vi "Measurement Logic.vi"() -> ()   [LabVIEW 2021, in "Line Regulation_PMIC.lvlib"]
uses:
  Line Regulation_PMIC.lvlib
  Measurement Configuration.ctl
  Measurement Results.ctl
  <vilib>/Plug-In SDKs/Measurements/Measure Call Context/Measure Call Context.lvclass
  <instrlib>/niDCPower/nidcpower.llb/niDCPower Sense.ctl
  <instrlib>/niDCPower/nidcpower.llb/niDCPower Source Mode.ctl
  <instrlib>/niDCPower/nidcpower.llb/niDCPower Wait For Event - Event.ctl
  <instrlib>/niDCPower/nidcpower.llb/niDCPower Output Function.ctl
  <instrlib>/niDCPower/nidcpower.llb/niDCPower Sequence Attribute Type.ctl
  <instrlib>/niDCPower/nidcpower.llb/niDCPower Get Channel Name From String.vi
  <instrlib>/niDCPower/nidcpower.llb/niDCPower Create Advanced Sequence Step With Channels.vi
  <instrlib>/niDCPower/nidcpower.llb/niDCPower Configure Digital Edge Source Trigger With Channels.vi
  <instrlib>/niDCPower/nidcpower.llb/niDCPower Configure Digital Edge Measure Trigger With Channels.vi
panel:
  out "measure call context out":refnum<class "Measure Call Context.lvclass">
  in  "measure call context in":refnum<class "Measure Call Context.lvclass">
  out "measurement results":T1
  in  "measurement configuration":T2={"Mode of operation"=enum."Perform measurement", "DUT setup time"=1.0, "Source delay"=0.005, "Aperture time"=0.005, "Nominal output voltage"=3.3, "Source resource name"="", "Source current limit"=25.0, "Source maximum power"=300.0, "Source sweep type"="Logarithmic", "Source start voltage"=6.0, "Source stop voltage"=20.0, "Source voltage sweep points/points per decade"=4, "Load resource name"="", "Load voltage limit range"=6.0, "Load current level"=0.1}
  out "error out":errorcluster
  in  "error in":errorcluster
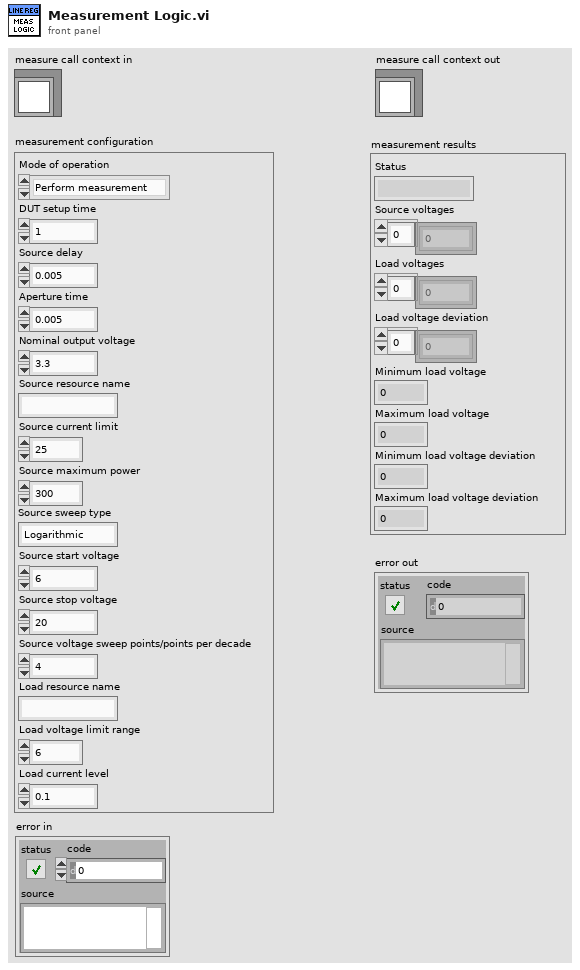
[diagram p1: front panel]
types:
  T1 = typedef "Line Regulation_PMIC.lvlib/Measurement Results.ctl" = cluster{"Status":string, "Source voltages":dbl[], "Load voltages":dbl[], "Load voltage deviation":dbl[], "Minimum load voltage":dbl, "Maximum load voltage":dbl, "Minimum load voltage deviation":dbl, "Maximum load voltage deviation":dbl}
  T2 = typedef "Line Regulation_PMIC.lvlib/Measurement Configuration.ctl" = cluster{"Mode of operation":enum32{"Power on the DUT", "Perform measurement", "Power off the DUT"}, "DUT setup time":dbl, "Source delay":dbl, "Aperture time":dbl, "Nominal output voltage":dbl, "Source resource name":string, "Source current limit":dbl, "Source maximum power":dbl, "Source sweep type":string, "Source start voltage":dbl, "Source stop voltage":dbl, "Source voltage sweep points/points per decade":i32, "Load resource name":string, "Load voltage limit range":dbl, "Load current level":dbl}
  T3 = cluster{"Voltage values":dbl[], "Source out":refnum<k15>, "Source channel name":string, "Load out":refnum<k15>, "Load channel name":string, "Source terminal name":string, "Measure terminal name":string, "Source sequence name":string, "Measurement Results":T1}
  T4 = enum32{"Power on the DUT", "Perform measurement", "Power off the DUT"}
  T5 = typedef "niDCPower Wait For Event - Event.ctl" = i32
  T6 = typedef "niDCPower Source Mode.ctl" = i32
  T7 = typedef "niDCPower Sense.ctl" = i32
  T8 = typedef "niDCPower Sequence Attribute Type.ctl" = i32
  T9 = typedef "niDCPower Output Function.ctl" = i32
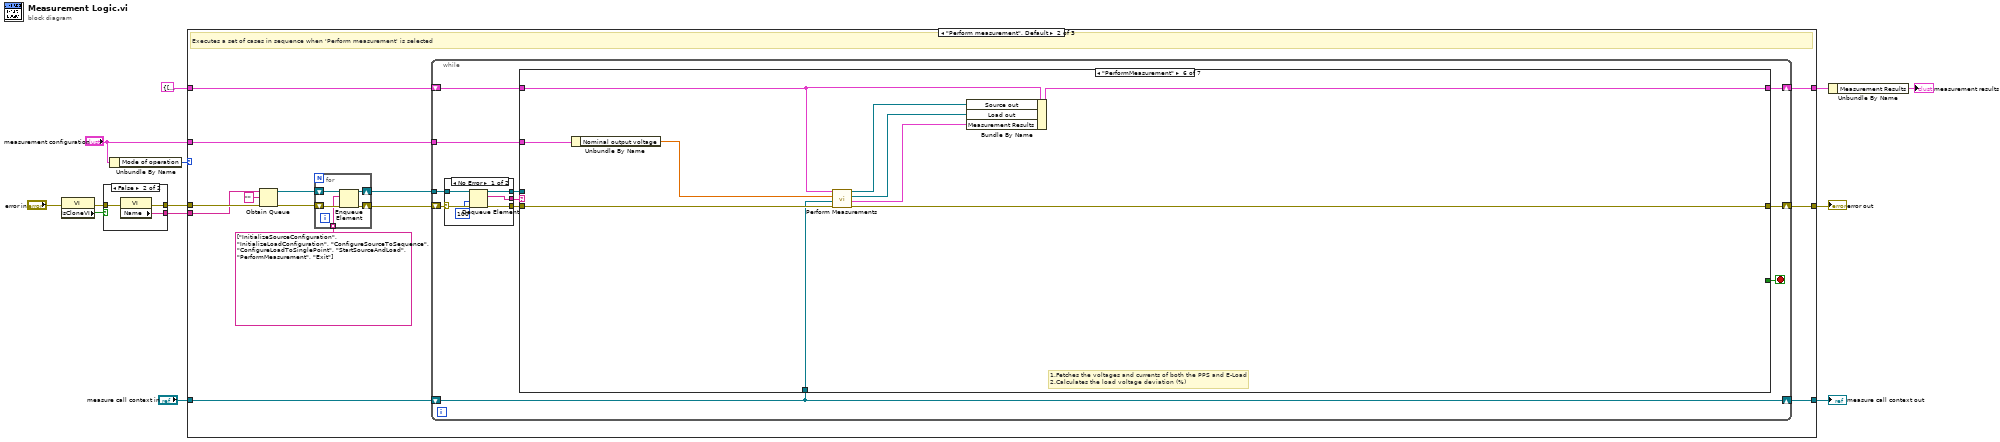
[diagram p0: block diagram]
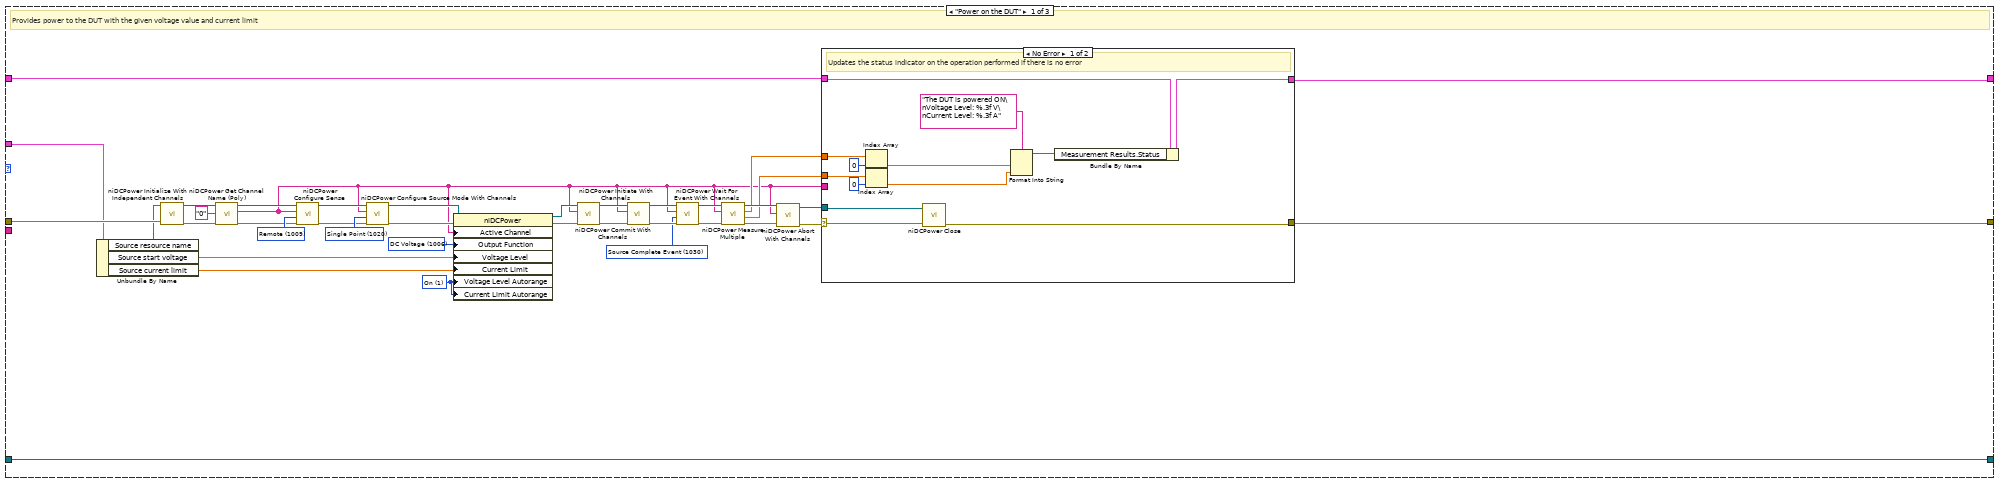
[diagram p2: hidden frame]
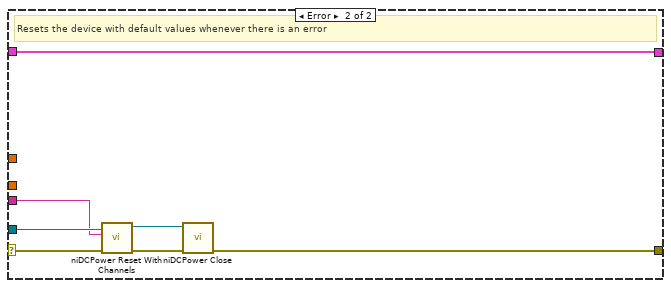
[diagram p3: hidden frame]
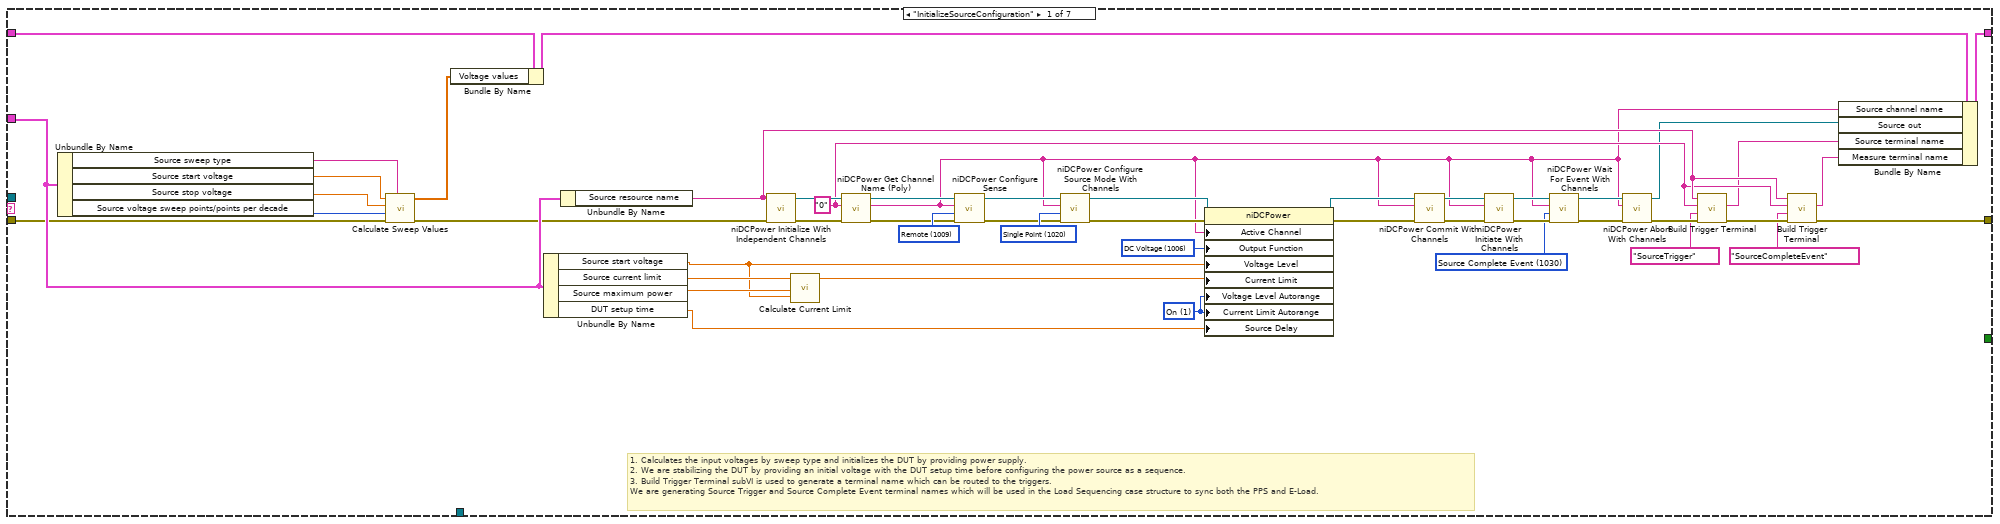
[diagram p4: hidden frame]
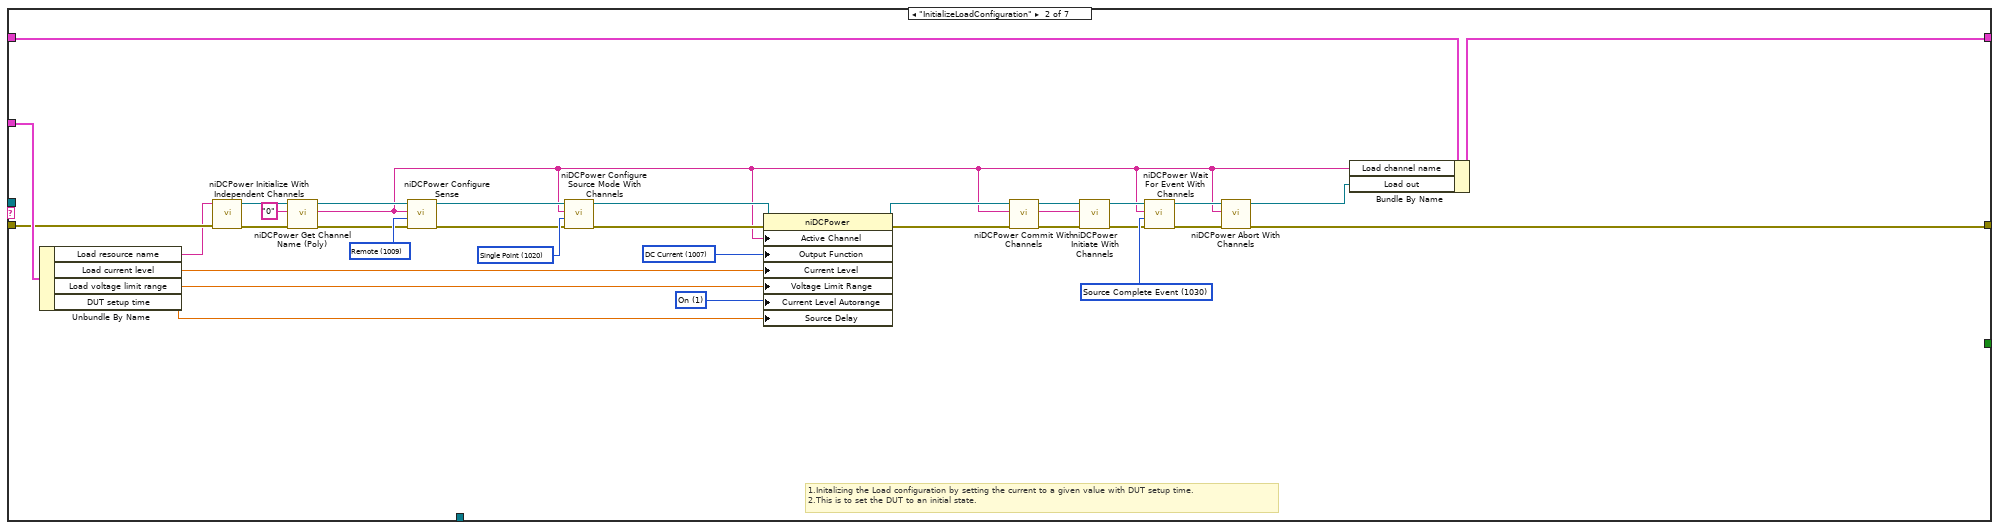
[diagram p5: hidden frame]
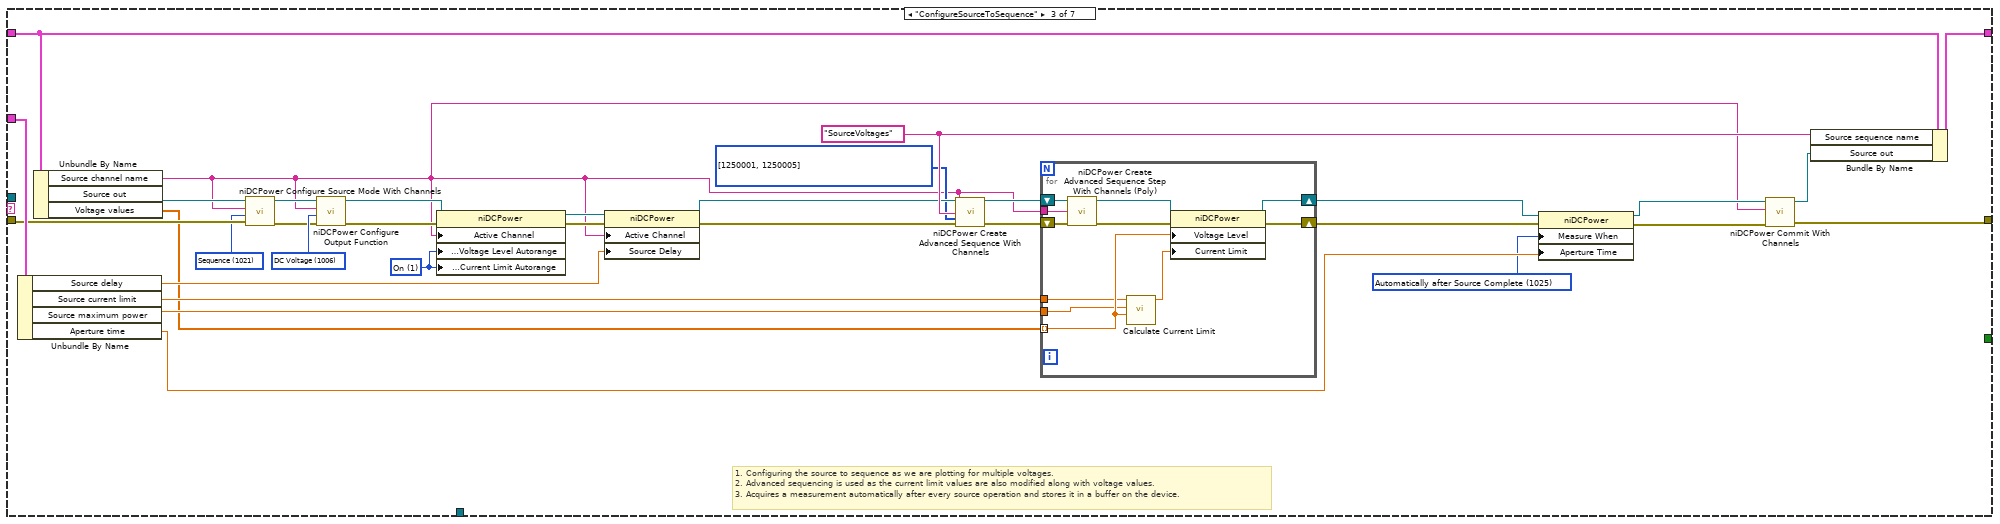
[diagram p6: hidden frame]
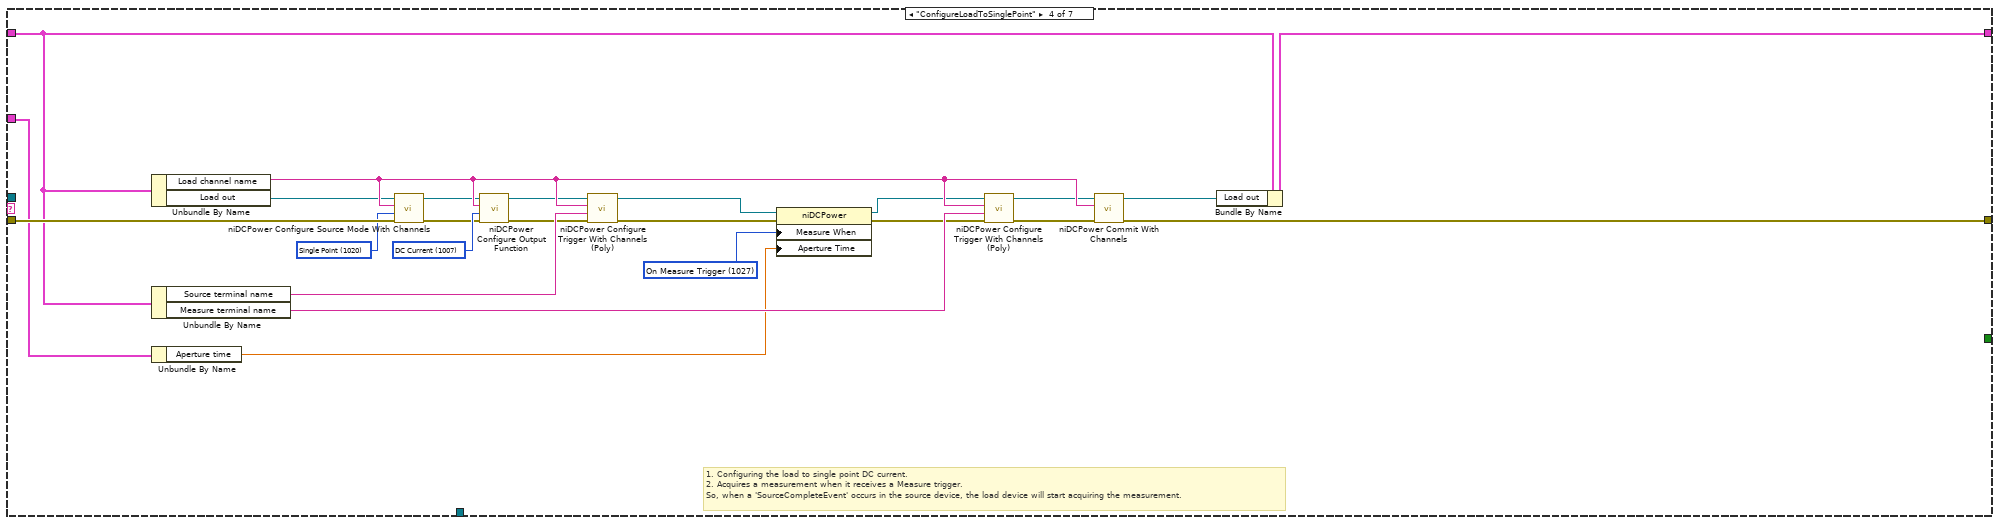
[diagram p7: hidden frame]
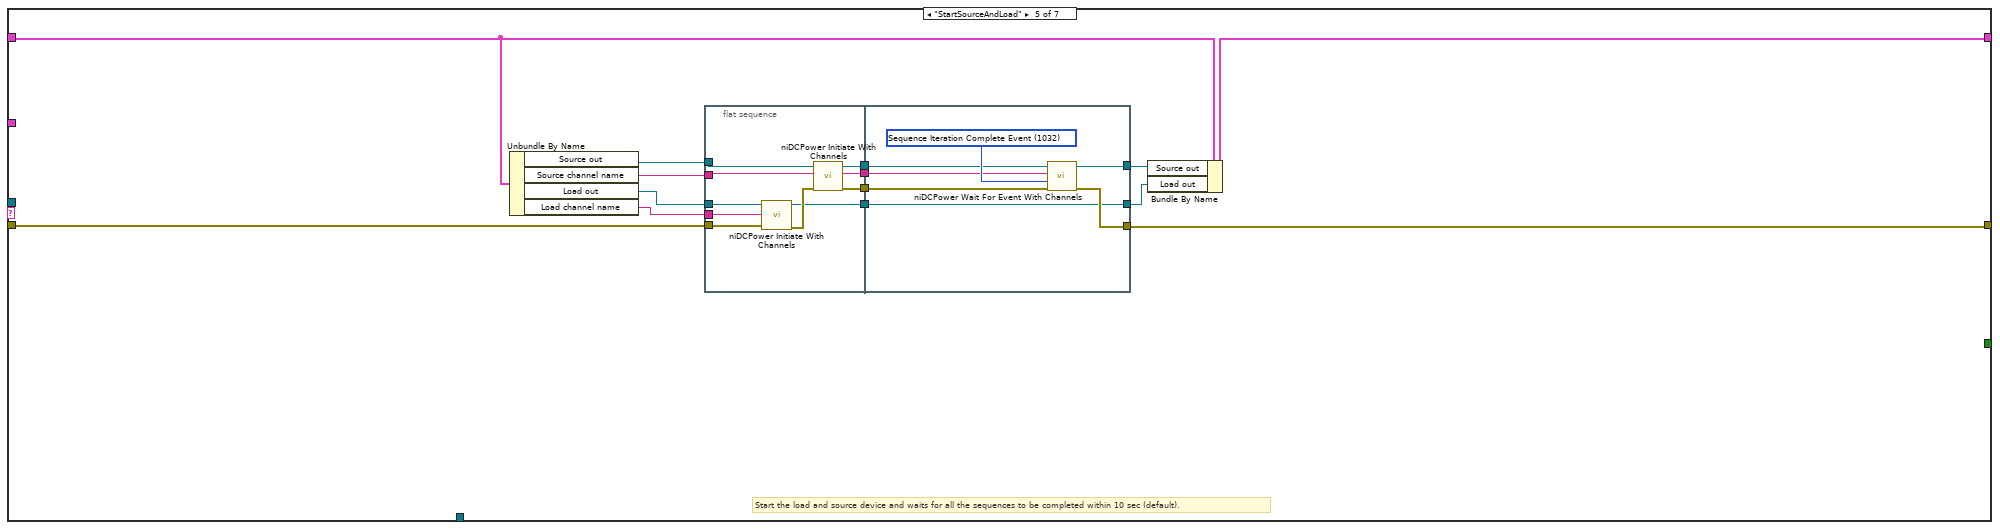
[diagram p8: hidden frame]
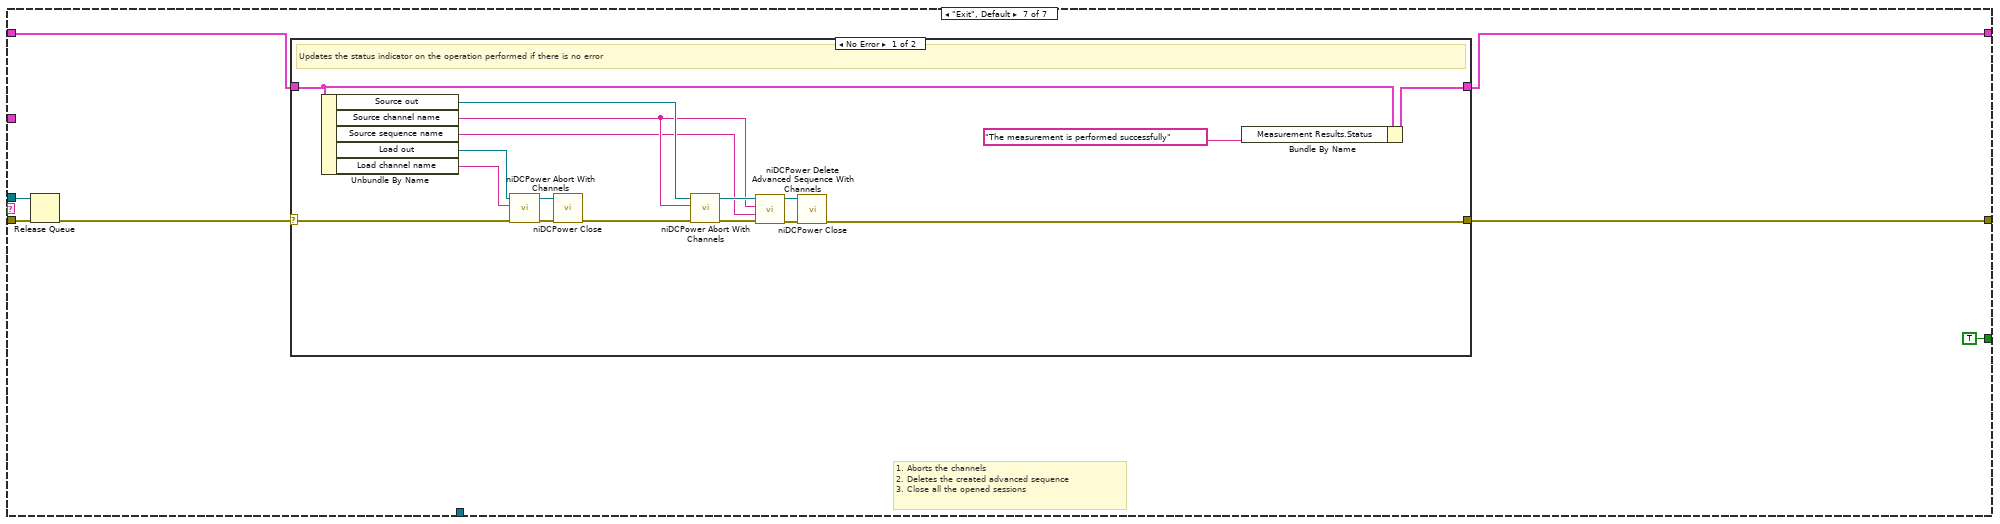
[diagram p9: hidden frame]
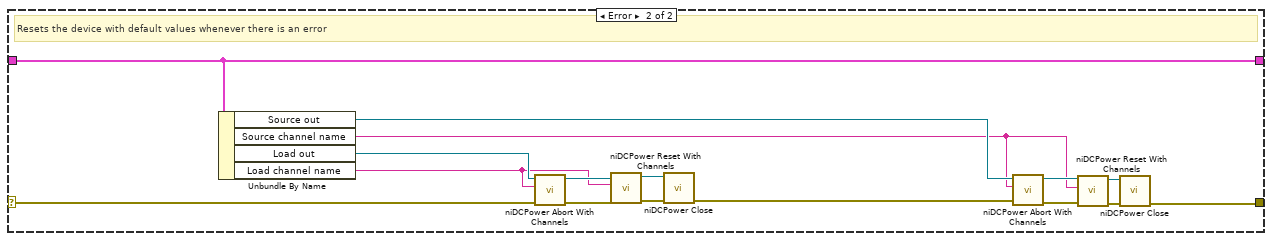
[diagram p10: hidden frame]
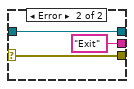
[diagram p11: hidden frame]
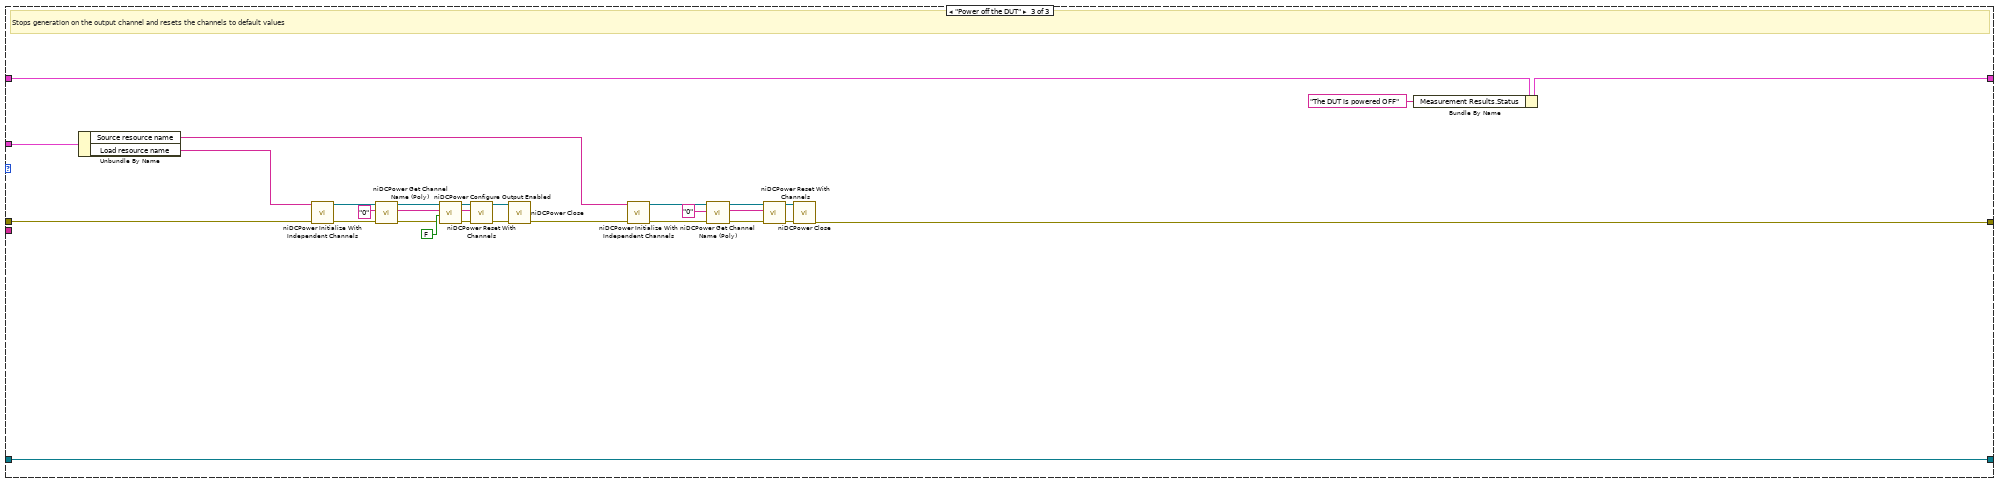
[diagram p12: hidden frame]
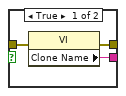
[diagram p13: hidden frame]
diagram:
  n1 = property class="VI"(error in="error in") -> (error out=w12:errorcluster, "IsCloneVI"=w13:bool)  [unwired: 1 in, 1 out]
  n2 = case shown="False" w13 {
    tunnel: [w16 w19] -> w9
    tunnel: [w15 w18] -> w8
    tunnel: w12 -> [w14 w17]
    frame True {
      n3 = property class="VI"(error in=w14) -> (error out=w16:errorcluster, "Clone Name"=w15:string)  [unwired: 1 in, 1 out]
    }
    frame False {
      n4 = property class="VI"(error in=w17) -> (error out=w19:errorcluster, "Name"=w18:string)  [unwired: 1 in, 1 out]
    }
  }
  n5 = Unbundle By Name("measurement configuration") -> ("Mode of operation"=w7:T4)
  n6 = case shown="\"Perform measurement\", Default" w7 {
    tunnel: w9 -> [w37 w87 w362]
    tunnel: w8 -> [_ w86 _]
    tunnel: "measurement configuration" -> [w30 w83 w350]
    tunnel: T3 {"Voltage values"=[], "Source out"="", "Source channel name"="", "Load out"="", "Load channel name"="", "Source terminal name"="", "Measure terminal name"="", "Source sequence name"="", "Measurement Results"={"Status"="", "Source voltages"=[], "Load voltages"=[], "Load voltage deviation"=[], "Minimum load voltage"=0.0, "Maximum load voltage"=0.0, "Minimum load voltage deviation"=0.0, "Maximum load voltage deviation"=0.0}} -> [w22 w82 w347]
    tunnel: "measure call context in" -> [w28 w80 w348]
    tunnel: [w28 w79 w348] -> w3
    tunnel: [w20 w78 w349] -> w2
    tunnel: [w21 w77 w345] -> w1
    frame "Power on the DUT" {
      w40 = 1 items=["Off", "On"] ("Source:DC Voltage:Voltage Level Autorange")
      w41 = T5 1030 items=["Source Complete Event"=1030, "Measure Complete Event"=1031, "Sequence Iteration Complete Event"=1032, "Sequence Engine Done Event"=1033, "Pulse Complete Event"=1051, "Ready For Pulse Trigger Event"=1052] ("event")
      w52 = T6 1020 items=["Single Point"=1020, "Sequence"=1021] ("source mode")
      w47 = 1006 items=["DC Voltage"=1006, "DC Current"=1007, "Pulse Voltage"=1049, "Pulse Current"=1050] ("Source:Output Function")
      w42 = T7 1009 items=["Local"=1008, "Remote"=1009] ("sense")
      # "Provides power to the DUT with the given voltage value and current limit"
      n7 = Unbundle By Name(w30) -> ("Source resource name"=w34:string, "Source start voltage"=w29:dbl, "Source current limit"=w35:dbl)
      n8 = call <instrlib>:"niDCPower Initialize With Independent Channels.vi"("error in (no error)"=w37, "resource name"=w34) -> ("error out"=w39:errorcluster, "instrument handle out"=w43:refnum<k15>)  [unwired: 8 in]
      n9 = call-poly <instrlib>:"niDCPower Get Channel Name (Poly).vi"("index"="0", "instrument handle"=w43) -> ("name"=w23:string, "instrument handle out"=w38:refnum<k15>)  [unwired: 7 in, 1 out]
      n10 = call <instrlib>:"niDCPower Configure Sense.vi"("error in (no error)"=w39, "sense"=w42, "channel name"=w23, "instrument handle"=w38) -> ("error out"=w50:errorcluster, "instrument handle out"=w48:refnum<k15>)  [unwired: 6 in]
      n11 = call <instrlib>:"niDCPower Configure Source Mode With Channels.vi"("error in (no error)"=w50, "source mode"=w52, "channel name"=w23, "instrument handle"=w48) -> ("error out"=w51:errorcluster, "instrument handle out"=w49:refnum<k15>)  [unwired: 6 in]
      n12 = property class="niDCPower"(reference=w49, error in=w51, "Active Channel"=w23, "Output Function"=w47, "Voltage Level"=w29, "Current Limit"=w35, "Voltage Level Autorange"=w40, "Current Limit Autorange"=w40) -> (reference out=w53:refnum<k15>, error out=w54:errorcluster)
      n13 = call <instrlib>:"niDCPower Commit With Channels.vi"("error in (no error)"=w54, "channel name"=w23, "instrument handle"=w53) -> ("error out"=w56:errorcluster, "instrument handle out"=w55:refnum<k15>)  [unwired: 7 in]
      n14 = call <instrlib>:"niDCPower Initiate With Channels.vi"("error in (no error)"=w56, "channel name"=w23, "instrument handle"=w55) -> ("error out"=w44:errorcluster, "instrument handle out"=w45:refnum<k15>)  [unwired: 7 in]
      n15 = call <instrlib>:"niDCPower Wait For Event With Channels.vi"("error in (no error)"=w44, "event"=w41, "channel name"=w23, "instrument handle"=w45) -> ("error out"=w32:errorcluster, "instrument handle out"=w46:refnum<k15>)  [unwired: 6 in]
      n16 = call <instrlib>:"niDCPower Measure Multiple.vi"("error in (no error)"=w32, "channel name"=w23, "instrument handle"=w46) -> ("error out"=w31:errorcluster, "current measurements"=w24:dbl[], "voltage measurements"=w25:dbl[], "instrument handle out"=w33:refnum<k15>)  [unwired: 5 in]
      n17 = call <instrlib>:"niDCPower Abort With Channels.vi"("error in (no error)"=w31, "channel name"=w23, "instrument handle"=w33) -> ("error out"=w27:errorcluster, "instrument handle out"=w26:refnum<k15>)  [unwired: 7 in]
      n18 = case shown="No Error" w27 {
        selector: w27 -> [w69 w74]
        tunnel: [w68 w73] -> w20
        tunnel: [w67 w70] -> w21
        tunnel: w26 -> [w62 w72]
        tunnel: w23 -> [_ w71]
        tunnel: w25 -> [w61 _]
        tunnel: w24 -> [w60 _]
        tunnel: w22 -> [w59 w70]
        frame No Error {
          # "Updates the status indicator on the operation performed if there is no error"
          n19 = Index Array(array=w61, index=0) -> (element=w58:dbl)
          n20 = Index Array(array=w60, index=0) -> (element=w57:dbl)
          n21 = call <instrlib>:"niDCPower Close.vi"("error in (no error)"=w69, "instrument handle"=w62) -> ("error out"=w68:errorcluster)  [unwired: 9 out]
          n22 = Format Into String(format string="The DUT is powered ON\nVoltage Level: %.3f V\nCurrent Level: %.3f A" ("message"), w58, w57) -> (resulting string=w65:string)  [unwired: 2 in, 1 out]
          n23 = Bundle By Name(cluster=w59, "Measurement Results.Status"=w65) -> (w67:T3)
        }
        frame Error {
          # "Resets the device with default values whenever there is an error"
          n24 = call <instrlib>:"niDCPower Reset With Channels.vi"("error in (no error)"=w74, "channel name"=w71, "instrument handle"=w72) -> ("error out"=w76:errorcluster, "instrument handle out"=w75:refnum<k15>)  [unwired: 7 in]
          n25 = call <instrlib>:"niDCPower Close.vi"("error in (no error)"=w76, "instrument handle"=w75) -> ("error out"=w73:errorcluster)  [unwired: 9 out]
        }
      }
    }
    frame "Perform measurement", Default {
      # "Executes a set of cases in sequence when 'Perform measurement' is selected"
      n26 = Obtain Queue(name (unnamed)=w86, element data type="", error in (no error)=w87) -> (queue out=w89:refnum<queue>, error out=w90:errorcluster)  [unwired: 2 in, 1 out]
      n27 = for {
        shift-right: [w342] -> w84
        shift-left: w89 -> [w344]
        shift-right: [w341] -> w81
        shift-left: w90 -> [w343]
        tunnel: string[] ["InitializeSourceConfiguration", "InitializeLoadConfiguration", "ConfigureSourceToSequence", "ConfigureLoadToSinglePoint", "StartSourceAndLoad", "PerformMeasurement", "Exit"] ("Step sequence") -> [w340] mode=indexing
        n28 = Enqueue Element(queue=w344, element=w340, error in (no error)=w343) -> (queue out=w342:refnum<queue>, error out=w341:errorcluster)  [unwired: 1 in, 1 out]
      }
      n29 = while {
        tunnel: w84 -> [w101]
        tunnel: w83 -> [w97]
        shift-right: [w94] -> w77
        shift-left: w82 -> [w95]
        shift-right: [w93] -> w78
        shift-left: w81 -> [w100]
        shift-right: [w92] -> w79
        shift-left: w80 -> [w92]
        stop <- w91 stop-if-true
        n30 = case shown="No Error" w100 {
          selector: w100 -> [w334 w338]
          tunnel: w101 -> [w336 w337]
          tunnel: [w335 "Exit" ("t")] -> w99
          tunnel: [w333 w338] -> w96
          tunnel: [w331 w337] -> w98
          frame No Error {
            n31 = Dequeue Element(queue=w336, timeout in ms (-1)=100, error in (no error)=w334) -> (queue out=w331:refnum<queue>, element=w335:string, error out=w333:errorcluster)  [unwired: 1 out]
          }
          frame Error {
          }
        }
        n32 = case shown="\"PerformMeasurement\"" w99 {
          tunnel: w98 -> [_ _ _ _ _ _ w296]
          tunnel: w97 -> [w128 w182 w213 w245 _ w289 _]
          tunnel: w96 -> [w120 w181 w212 w250 w257 w287 w295]
          tunnel: w95 -> [w148 w158 w215 w241 w256 w281 w292]
          tunnel: [w149 w178 w214 w240 w253 w290 w291] -> w94
          tunnel: [w111 w180 w205 w243 w252 w288 w294] -> w93
          tunnel: w92 -> [_ _ _ _ _ w285 _]
          tunnel: [_ _ _ _ _ _ TRUE] -> w91
          frame "InitializeSourceConfiguration" {
            w107 = "0" ("index")
            w130 = 1 items=["Off", "On"] ("Source:DC Voltage:Voltage Level Autorange")
            w131 = T5 1030 items=["Source Complete Event"=1030, "Measure Complete Event"=1031, "Sequence Iteration Complete Event"=1032, "Sequence Engine Done Event"=1033, "Pulse Complete Event"=1051, "Ready For Pulse Trigger Event"=1052] ("event")
            w143 = T6 1020 items=["Single Point"=1020, "Sequence"=1021] ("source mode")
            w138 = 1006 items=["DC Voltage"=1006, "DC Current"=1007, "Pulse Voltage"=1049, "Pulse Current"=1050] ("Source:Output Function")
            w132 = T7 1009 items=["Local"=1008, "Remote"=1009] ("sense")
            # "1. Calculates the input voltages by sweep type and initializes the DUT by providing power supply.\n2. We are stabilizing the DUT by providing an initial voltage with the DUT setup time before configuring the power source as a sequence.\n3. Build Trigger Terminal subVI is used to generate a terminal name which can be routed to the triggers.\nWe are generating Source Trigger and Source Complete Event terminal names which will be used in the Load Sequencing case structure to sync both the PPS and E-Load."
            n33 = Unbundle By Name(w128) -> ("Source sweep type"=w114:string, "Source start voltage"=w123:dbl, "Source stop voltage"=w122:dbl, "Source voltage sweep points/points per decade"=w121:i32)
            n34 = call "Calculate Sweep Values.vi"("Sweep type"=w114, "error in"=w120, "Points"=w121, "Stop level"=w122, "Start level"=w123) -> ("error out"=w119:errorcluster, "Sweep values"=w118:dbl[])  [unwired: 4 in, 1 out]
            n35 = Bundle By Name(cluster=w148, "Voltage values"=w118) -> (w127:T3)
            n36 = Unbundle By Name(w128) -> ("Source start voltage"=w102:dbl, "Source current limit"=w117:dbl, "Source maximum power"=w116:dbl, "DUT setup time"=w129:dbl)
            n37 = Unbundle By Name(w128) -> ("Source resource name"=w108:string)
            n38 = call <instrlib>:"niDCPower Initialize With Independent Channels.vi"("error in (no error)"=w119, "resource name"=w108) -> ("error out"=w125:errorcluster, "instrument handle out"=w133:refnum<k15>)  [unwired: 8 in]
            n39 = call "Calculate Current Limit.vi"("Voltage value"=w102, "Maximum power"=w116, "Current limit in"=w117) -> ("Current limit out"=w115:dbl)  [unwired: 8 in]
            n40 = call-poly <instrlib>:"niDCPower Get Channel Name (Poly).vi"("error in (no error)"=w125, "index"=w107, "instrument handle"=w133) -> ("error out"=w124:errorcluster, "name"=w104:string, "instrument handle out"=w126:refnum<k15>)  [unwired: 6 in]
            n41 = call <instrlib>:"niDCPower Configure Sense.vi"("error in (no error)"=w124, "sense"=w132, "channel name"=w104, "instrument handle"=w126) -> ("error out"=w141:errorcluster, "instrument handle out"=w139:refnum<k15>)  [unwired: 6 in]
            n42 = call <instrlib>:"niDCPower Configure Source Mode With Channels.vi"("error in (no error)"=w141, "source mode"=w143, "channel name"=w104, "instrument handle"=w139) -> ("error out"=w142:errorcluster, "instrument handle out"=w140:refnum<k15>)  [unwired: 6 in]
            n43 = property class="niDCPower"(reference=w140, error in=w142, "Active Channel"=w104, "Output Function"=w138, "Voltage Level"=w102, "Current Limit"=w115, "Voltage Level Autorange"=w130, "Current Limit Autorange"=w130, "Source Delay"=w129) -> (reference out=w144:refnum<k15>, error out=w145:errorcluster)
            n44 = call <instrlib>:"niDCPower Commit With Channels.vi"("error in (no error)"=w145, "channel name"=w104, "instrument handle"=w144) -> ("error out"=w147:errorcluster, "instrument handle out"=w146:refnum<k15>)  [unwired: 7 in]
            n45 = call <instrlib>:"niDCPower Initiate With Channels.vi"("error in (no error)"=w147, "channel name"=w104, "instrument handle"=w146) -> ("error out"=w134:errorcluster, "instrument handle out"=w135:refnum<k15>)  [unwired: 7 in]
            n46 = call <instrlib>:"niDCPower Wait For Event With Channels.vi"("error in (no error)"=w134, "event"=w131, "channel name"=w104, "instrument handle"=w135) -> ("error out"=w137:errorcluster, "instrument handle out"=w136:refnum<k15>)  [unwired: 6 in]
            n47 = call <instrlib>:"niDCPower Abort With Channels.vi"("error in (no error)"=w137, "channel name"=w104, "instrument handle"=w136) -> ("error out"=w113:errorcluster, "instrument handle out"=w103:refnum<k15>)  [unwired: 7 in]
            n48 = call "Build Trigger Terminal.vi"("error in (no error)"=w113, "Trigger/Event Name"="SourceTrigger", "Channel Name"=w107, "Resource Name"=w108) -> ("error out"=w112:errorcluster, "Terminal Name"=w106:string)  [unwired: 6 in]
            n49 = call "Build Trigger Terminal.vi"("error in (no error)"=w112, "Trigger/Event Name"="SourceCompleteEvent", "Channel Name"=w107, "Resource Name"=w108) -> ("error out"=w111:errorcluster, "Terminal Name"=w105:string)  [unwired: 6 in]
            n50 = Bundle By Name(cluster=w127, "Source channel name"=w104, "Source out"=w103, "Source terminal name"=w106, "Measure terminal name"=w105) -> (w149:T3)
          }
          frame "InitializeLoadConfiguration" {
            w173 = T6 1020 items=["Single Point"=1020, "Sequence"=1021] ("source mode")
            w166 = T5 1030 items=["Source Complete Event"=1030, "Measure Complete Event"=1031, "Sequence Iteration Complete Event"=1032, "Sequence Engine Done Event"=1033, "Pulse Complete Event"=1051, "Ready For Pulse Trigger Event"=1052] ("event")
            w160 = 1 items=["Off", "On"] ("Source:DC Current:Current Level Autorange")
            w162 = 1007 items=["DC Voltage"=1006, "DC Current"=1007, "Pulse Voltage"=1049, "Pulse Current"=1050] ("Source:Output Function")
            w161 = T7 1009 items=["Local"=1008, "Remote"=1009] ("sense")
            # "1.Initalizing the Load configuration by setting the current to a given value with DUT setup time.\n2.This is to set the DUT to an initial state."
            n51 = Unbundle By Name(w182) -> ("Load resource name"=w179:string, "Load current level"=w151:dbl, "Load voltage limit range"=w150:dbl, "DUT setup time"=w159:dbl)
            n52 = call <instrlib>:"niDCPower Initialize With Independent Channels.vi"("error in (no error)"=w181, "resource name"=w179) -> ("error out"=w155:errorcluster, "instrument handle out"=w163:refnum<k15>)  [unwired: 8 in]
            n53 = call-poly <instrlib>:"niDCPower Get Channel Name (Poly).vi"("error in (no error)"=w155, "index"="0", "instrument handle"=w163) -> ("error out"=w154:errorcluster, "name"=w153:string, "instrument handle out"=w157:refnum<k15>)  [unwired: 6 in]
            n54 = call <instrlib>:"niDCPower Configure Sense.vi"("error in (no error)"=w154, "sense"=w161, "channel name"=w153, "instrument handle"=w157) -> ("error out"=w170:errorcluster, "instrument handle out"=w169:refnum<k15>)  [unwired: 6 in]
            n55 = call <instrlib>:"niDCPower Configure Source Mode With Channels.vi"("error in (no error)"=w170, "source mode"=w173, "channel name"=w153, "instrument handle"=w169) -> ("error out"=w172:errorcluster, "instrument handle out"=w171:refnum<k15>)  [unwired: 6 in]
            n56 = property class="niDCPower"(reference=w171, error in=w172, "Active Channel"=w153, "Output Function"=w162, "Current Level"=w151, "Voltage Limit Range"=w150, "Current Level Autorange"=w160, "Source Delay"=w159) -> (reference out=w174:refnum<k15>, error out=w175:errorcluster)
            n57 = call <instrlib>:"niDCPower Commit With Channels.vi"("error in (no error)"=w175, "channel name"=w153, "instrument handle"=w174) -> ("error out"=w176:errorcluster, "instrument handle out"=w177:refnum<k15>)  [unwired: 7 in]
            n58 = call <instrlib>:"niDCPower Initiate With Channels.vi"("error in (no error)"=w176, "channel name"=w153, "instrument handle"=w177) -> ("error out"=w164:errorcluster, "instrument handle out"=w165:refnum<k15>)  [unwired: 7 in]
            n59 = call <instrlib>:"niDCPower Wait For Event With Channels.vi"("error in (no error)"=w164, "event"=w166, "channel name"=w153, "instrument handle"=w165) -> ("error out"=w168:errorcluster, "instrument handle out"=w167:refnum<k15>)  [unwired: 6 in]
            n60 = call <instrlib>:"niDCPower Abort With Channels.vi"("error in (no error)"=w168, "channel name"=w153, "instrument handle"=w167) -> ("error out"=w180:errorcluster, "instrument handle out"=w152:refnum<k15>)  [unwired: 7 in]
            n61 = Bundle By Name(cluster=w158, "Load channel name"=w153, "Load out"=w152) -> (w178:T3)
          }
          frame "ConfigureSourceToSequence" {
            w189 = 1025 items=["Automatically after Source Complete"=1025, "On Demand"=1026, "On Measure Trigger"=1027] ("Measurement:Advanced:Measure When")
            w197 = 1 items=["Off", "On"] ("DC Voltage:Voltage Level Autorange")
            w196 = T8[] [1250001, 1250005] items=["Source -> Output Function"=1150008, "Source -> Output Enabled"=1250006, "Source -> Output Resistance"=1150061, "Source -> Transient Response"=1150062, "Source -> Custom Transient Response -> Voltage Gain Bandwidth"=1150067, "Source -> Custom Transient Response -> Voltage Compensation Frequency"=1150068, "Source -> Custom Transient Response -> Voltage Pole-Zero Ratio"=1150069, "Source -> Custom Transient Response -> Current Gain Bandwidth"=1150070, "Source -> Custom Transient Response -> Current Compensation Frequency"=1150071, "Source -> Custom Transient Response -> Current Pole-Zero Ratio"=1150072, "Source -> DC Voltage -> Voltage Level"=1250001, "Source -> DC Voltage -> Voltage Level Range"=1150005, "Source -> DC Voltage -> Current Limit"=1250005, "Source -> DC Voltage -> Current Limit High"=1150187, "Source -> DC Voltage -> Current Limit Low"=1150188, "Source -> DC Voltage -> Current Limit Range"=1150004, "Source -> DC Current -> Current Level"=1150009, "Source -> DC Current -> Current Level Range"=1150011, "Source -> DC Current -> Voltage Limit"=1150010, "Source -> DC Current -> Voltage Limit High"=1150185, "Source -> DC Current -> Voltage Limit Low"=1150186, "Source -> DC Current -> Voltage Limit Range"=1150012, "Source -> Pulse Voltage -> Pulse Voltage Level"=1150080, "Source -> Pulse Voltage -> Pulse Bias Voltage Level"=1150082, "Source -> Pulse Voltage -> Pulse Voltage Level Range"=1150084, "Source -> Pulse Voltage -> Pulse Current Limit"=1150081, "Source -> Pulse Voltage -> Pulse Current Limit High"=1150193, "Source -> Pulse Voltage -> Pulse Current Limit Low"=1150194, "Source -> Pulse Voltage -> Pulse Bias Current Limit"=1150083, "Source -> Pulse Voltage -> Pulse Bias Current Limit High"=1150195, "Source -> Pulse Voltage -> Pulse Bias Current Limit Low"=1150196, "Source -> Pulse Voltage -> Pulse Current Limit Range"=1150085, "Source -> Pulse Current -> Pulse Current Level"=1150086, "Source -> Pulse Current -> Pulse Bias Current Level"=1150088, "Source -> Pulse Current -> Pulse Current Level Range"=1150090, "Source -> Pulse Current -> Pulse Voltage Limit"=1150087, "Source -> Pulse Current -> Pulse Voltage Limit High"=1150189, "Source -> Pulse Current -> Pulse Voltage Limit Low"=1150190, "Source -> Pulse Current -> Pulse Bias Voltage Limit"=1150089, "Source -> Pulse Current -> Pulse Bias Voltage Limit High"=1150191, "Source -> Pulse Current -> Pulse Bias Voltage Limit Low"=1150192, "Source -> Pulse Current -> Pulse Voltage Limit Range"=1150091, "Source -> Advanced -> Source Delay"=1150051, "Source -> Advanced -> Pulse Bias Delay"=1150092, "Source -> Advanced -> Pulse On Time"=1150093, "Source -> Advanced -> Pulse Off Time"=1150094, "Source -> Advanced -> OVP Enabled"=1250002, "Source -> Advanced -> OVP Limit"=1250003, "Source -> Advanced -> Compliance Limit Symmetry"=1150184, "Source -> Advanced -> Sequence Step Delta Time"=1150198, "Measurement -> Sense"=1150013, "Measurement -> Aperture Time"=1150058, "Measurement -> Measure Record Length"=1150063, "Measurement -> Advanced -> DC Noise Rejection"=1150066, "Measurement -> Autorange"=1150244, "Measurement -> Advanced -> Autorange Behavior"=1150245, "Measurement -> Advanced -> Autorange Aperture Time Mode"=1150246, "Measurement -> Advanced -> Autorange Minimum Aperture Time"=1150247, "Measurement -> Advanced -> Autorange Minimum Aperture Time Units"=1150248, "Measurement -> Advanced -> Autorange Minimum Current Range"=1150255, "Measurement -> Advanced -> Autorange Minimum Voltage Range"=1150256, "Measurement -> Advanced -> Autorange Threshold Mode"=1150257, "Measurement -> Advanced -> Autorange Maximum Delay After Range Change"=1150322, "LCR -> Instrument Mode"=1150208, "LCR -> LCR Stimulus Function"=1150209, "LCR -> LCR Frequency"=1150210, "LCR -> LCR Voltage Amplitude"=1150211, "LCR -> LCR Current Amplitude"=1150212, "LCR -> LCR DC Bias Source"=1150213, "LCR -> LCR DC Bias Voltage Level"=1150214, "LCR -> LCR DC Bias Current Level"=1150215, "LCR -> LCR Impedance Autorange"=1150216, "LCR -> LCR Impedance Range"=1150217, "LCR -> LCR Measurement Time"=1150218, "LCR -> LCR Custom Measurement Time"=1150258, "LCR -> LCR Source Delay Mode"=1150315, "LCR -> Compensation -> Open -> Enabled"=1150220, "LCR -> Compensation -> Open -> Conductance"=1150261, "LCR -> Compensation -> Open -> Susceptance"=1150262, "LCR -> Compensation -> Short -> Enabled"=1150221, "LCR -> Compensation -> Short -> Resistance"=1150263, "LCR -> Compensation -> Short -> Reactance"=1150264, "LCR -> Compensation -> Load -> Enabled"=1150222, "LCR -> Compensation -> Load -> Measured Resistance"=1150268, "LCR -> Compensation -> Load -> Measured Reactance"=1150269, "LCR -> Compensation -> Load -> Actual Resistance"=1150270, "LCR -> Compensation -> Load -> Actual Reactance"=1150271] ("advanced sequence properties")
            w204 = "SourceVoltages" ("sequence name")
            w193 = T9 1006 items=["DC Voltage"=1006, "DC Current"=1007, "Pulse Voltage"=1049, "Pulse Current"=1050] ("output function")
            w192 = T6 1021 items=["Single Point"=1020, "Sequence"=1021] ("source mode")
            # "1. Configuring the source to sequence as we are plotting for multiple voltages.\n2. Advanced sequencing is used as the current limit values are also modified along with voltage values.\n3. Acquires a measurement automatically after every source operation and stores it in a buffer on the device."
            n62 = Unbundle By Name(w213) -> ("Source delay"=w211:dbl, "Source current limit"=w210:dbl, "Source maximum power"=w209:dbl, "Aperture time"=w208:dbl)
            n63 = Unbundle By Name(w215) -> ("Source channel name"=w183:string, "Source out"=w207:refnum<k15>, "Voltage values"=w206:dbl[])
            n64 = call <instrlib>:"niDCPower Configure Source Mode With Channels.vi"("error in (no error)"=w212, "source mode"=w192, "channel name"=w183, "instrument handle"=w207) -> ("error out"=w190:errorcluster, "instrument handle out"=w191:refnum<k15>)  [unwired: 6 in]
            n65 = call <instrlib>:"niDCPower Configure Output Function.vi"("error in (no error)"=w190, "output function"=w193, "channel name"=w183, "instrument handle"=w191) -> ("error out"=w201:errorcluster, "instrument handle out"=w200:refnum<k15>)  [unwired: 6 out]
            n66 = property class="niDCPower"(reference=w200, error in=w201, "Active Channel"=w183, "Source:DC Voltage:Voltage Level Autorange"=w197, "Source:DC Voltage:Current Limit Autorange"=w197) -> (reference out=w198:refnum<k15>, error out=w199:errorcluster)
            n67 = property class="niDCPower"(reference=w198, error in=w199, "Active Channel"=w183, "Source Delay"=w211) -> (reference out=w202:refnum<k15>, error out=w203:errorcluster)
            n68 = call <instrlib>:"niDCPower Create Advanced Sequence With Channels.vi"("instrument handle"=w202, "channel name"=w183, "sequence name"=w204, "advanced sequence properties"=w196, "error in (no error)"=w203) -> ("instrument handle out"=w194:refnum<k15>, "error out"=w195:errorcluster)  [unwired: 9 in]
            n69 = for {
              shift-right: [w223] -> w184
              shift-left: w195 -> [w226]
              shift-right: [w222] -> w185
              shift-left: w194 -> [w221]
              tunnel: w209 -> [w218]
              tunnel: w206 -> [w219] mode=indexing
              tunnel: w210 -> [w217]
              tunnel: w183 -> [w220]
              n70 = call-poly <instrlib>:"niDCPower Create Advanced Sequence Step With Channels (Poly).vi"("error in (no error)"=w226, "channel name"=w220, "instrument handle"=w221) -> ("error out"=w224:errorcluster, "instrument handle out"=w225:refnum<k15>)  [unwired: 7 in]
              n71 = call "Calculate Current Limit.vi"("Voltage value"=w219, "Maximum power"=w218, "Current limit in"=w217) -> ("Current limit out"=w216:dbl)  [unwired: 8 in]
              n72 = property class="niDCPower"(reference=w225, error in=w224, "Voltage Level"=w219, "Current Limit"=w216) -> (reference out=w222:refnum<k15>, error out=w223:errorcluster)
            }
            n73 = property class="niDCPower"(reference=w185, error in=w184, "Measure When"=w189, "Aperture Time"=w208) -> (reference out=w187:refnum<k15>, error out=w188:errorcluster)
            n74 = call <instrlib>:"niDCPower Commit With Channels.vi"("error in (no error)"=w188, "channel name"=w183, "instrument handle"=w187) -> ("error out"=w205:errorcluster, "instrument handle out"=w186:refnum<k15>)  [unwired: 7 in]
            n75 = Bundle By Name(cluster=w215, "Source sequence name"=w204, "Source out"=w186) -> (w214:T3)
          }
          frame "ConfigureLoadToSinglePoint" {
            w234 = T9 1007 items=["DC Voltage"=1006, "DC Current"=1007, "Pulse Voltage"=1049, "Pulse Current"=1050] ("output function")
            w233 = 1027 items=["Automatically after Source Complete"=1025, "On Demand"=1026, "On Measure Trigger"=1027] ("Measurement:Advanced:Measure When")
            w232 = T6 1020 items=["Single Point"=1020, "Sequence"=1021] ("source mode")
            # "1. Configuring the load to single point DC current.\n2. Acquires a measurement when it receives a Measure trigger. \nSo, when a 'SourceCompleteEvent' occurs in the source device, the load device will start acquiring the measurement."
            n76 = Unbundle By Name(w241) -> ("Load channel name"=w249:string, "Load out"=w248:refnum<k15>)
            n77 = Unbundle By Name(w241) -> ("Source terminal name"=w247:string, "Measure terminal name"=w246:string)
            n78 = Unbundle By Name(w245) -> ("Aperture time"=w244:dbl)
            n79 = call <instrlib>:"niDCPower Configure Source Mode With Channels.vi"("error in (no error)"=w250, "source mode"=w232, "channel name"=w249, "instrument handle"=w248) -> ("error out"=w230:errorcluster, "instrument handle out"=w231:refnum<k15>)  [unwired: 6 in]
            n80 = call <instrlib>:"niDCPower Configure Output Function.vi"("error in (no error)"=w230, "output function"=w234, "channel name"=w249, "instrument handle"=w231) -> ("error out"=w238:errorcluster, "instrument handle out"=w237:refnum<k15>)  [unwired: 6 out]
            n81 = call-poly <instrlib>:"niDCPower Configure Trigger With Channels (Poly).vi"("error in (no error)"=w238, "input terminal"=w247, "channel name"=w249, "instrument handle"=w237) -> ("error out"=w227:errorcluster, "instrument handle out"=w239:refnum<k15>)  [unwired: 6 in]
            n82 = property class="niDCPower"(reference=w239, error in=w227, "Measure When"=w233, "Aperture Time"=w244) -> (reference out=w229:refnum<k15>, error out=w228:errorcluster)
            n83 = call-poly <instrlib>:"niDCPower Configure Trigger With Channels (Poly).vi"("error in (no error)"=w228, "input terminal"=w246, "channel name"=w249, "instrument handle"=w229) -> ("error out"=w235:errorcluster, "instrument handle out"=w236:refnum<k15>)  [unwired: 6 in]
            n84 = call <instrlib>:"niDCPower Commit With Channels.vi"("error in (no error)"=w235, "channel name"=w249, "instrument handle"=w236) -> ("error out"=w243:errorcluster, "instrument handle out"=w242:refnum<k15>)  [unwired: 7 in]
            n85 = Bundle By Name(cluster=w241, "Load out"=w242) -> (w240:T3)
          }
          frame "StartSourceAndLoad" {
            # "Start the load and source device and waits for all the sequences to be completed within 10 sec (default)."
            n86 = Unbundle By Name(w256) -> ("Source out"=w261:refnum<k15>, "Source channel name"=w258:string, "Load out"=w260:refnum<k15>, "Load channel name"=w259:string)
            n87 = flat-sequence {
              tunnel: [w272] -> w264
              tunnel: [w271] -> w263
              tunnel: [w270] -> w262
              tunnel: w257 -> [w269]
              tunnel: w260 -> [w268]
              tunnel: w261 -> [w267]
              tunnel: w258 -> [w265]
              tunnel: w259 -> [w266]
              tunnel: [w265] -> w251
              tunnel: w264 -> [w279]
              tunnel: w263 -> [w278]
              tunnel: w262 -> [w275]
              tunnel: [w276] -> w255
              tunnel: [w277] -> w252
              tunnel: [w275] -> w254
              tunnel: w251 -> [w274]
              frame #0 {
                n88 = call <instrlib>:"niDCPower Initiate With Channels.vi"("error in (no error)"=w269, "channel name"=w266, "instrument handle"=w268) -> ("error out"=w273:errorcluster, "instrument handle out"=w270:refnum<k15>)  [unwired: 7 in]
                n89 = call <instrlib>:"niDCPower Initiate With Channels.vi"("error in (no error)"=w273, "channel name"=w265, "instrument handle"=w267) -> ("error out"=w271:errorcluster, "instrument handle out"=w272:refnum<k15>)  [unwired: 7 in]
              }
              frame #1 {
                w280 = T5 1032 items=["Source Complete Event"=1030, "Measure Complete Event"=1031, "Sequence Iteration Complete Event"=1032, "Sequence Engine Done Event"=1033] ("event")
                n90 = call <instrlib>:"niDCPower Wait For Event With Channels.vi"("error in (no error)"=w278, "event"=w280, "channel name"=w274, "instrument handle"=w279) -> ("error out"=w277:errorcluster, "instrument handle out"=w276:refnum<k15>)  [unwired: 6 in]
              }
            }
            n91 = Bundle By Name(cluster=w256, "Source out"=w255, "Load out"=w254) -> (w253:T3)
          }
          frame "PerformMeasurement" {
            # "1.Fetches the voltages and currents of both the PPS and E-Load\n2.Calculates the load voltage deviation (%)"
            n92 = Unbundle By Name(w289) -> ("Nominal output voltage"=w286:dbl)
            n93 = call "Perform Measurements.vi"("error in"=w287, "Measurement Context"=w285, "Nominal output voltage"=w286, "Reference values"=w281) -> ("error out"=w288:errorcluster, "Measurement Results"=w282:T1, "Load out"=w283:refnum<k15>, "Source out"=w284:refnum<k15>)  [unwired: 4 in]
            n94 = Bundle By Name(cluster=w281, "Source out"=w284, "Load out"=w283, "Measurement Results"=w282) -> (w290:T3)
          }
          frame "Exit", Default {
            # "1. Aborts the channels\n2. Deletes the created advanced sequence\n3. Close all the opened sessions"
            n95 = Release Queue(queue=w296, error in (no error)=w295) -> (error out=w293:errorcluster)  [unwired: 1 in, 2 out]
            n96 = case shown="No Error" w293 {
              selector: w293 -> [w299 w330]
              tunnel: [w298 w329] -> w294
              tunnel: w292 -> [w300 w328]
              tunnel: [w313 w328] -> w291
              frame No Error {
                # "Updates the status indicator on the operation performed if there is no error"
                n97 = Unbundle By Name(w300) -> ("Source out"=w311:refnum<k15>, "Source channel name"=w305:string, "Source sequence name"=w301:string, "Load out"=w310:refnum<k15>, "Load channel name"=w309:string)
                n98 = call <instrlib>:"niDCPower Abort With Channels.vi"("error in (no error)"=w299, "channel name"=w309, "instrument handle"=w310) -> ("error out"=w312:errorcluster, "instrument handle out"=w302:refnum<k15>)  [unwired: 7 in]
                n99 = call <instrlib>:"niDCPower Close.vi"("error in (no error)"=w312, "instrument handle"=w302) -> ("error out"=w304:errorcluster)  [unwired: 9 in]
                n100 = call <instrlib>:"niDCPower Abort With Channels.vi"("error in (no error)"=w304, "channel name"=w305, "instrument handle"=w311) -> ("error out"=w307:errorcluster, "instrument handle out"=w306:refnum<k15>)  [unwired: 7 in]
                n101 = call <instrlib>:"niDCPower Delete Advanced Sequence With Channels.vi"("error in (no error)"=w307, "sequence name"=w301, "channel name"=w305, "instrument handle"=w306) -> ("error out"=w308:errorcluster, "instrument handle out"=w303:refnum<k15>)  [unwired: 6 in]
                n102 = call <instrlib>:"niDCPower Close.vi"("error in (no error)"=w308, "instrument handle"=w303) -> ("error out"=w298:errorcluster)  [unwired: 9 in]
                n103 = Bundle By Name(cluster=w300, "Measurement Results.Status"="The measurement is performed successfully" ("message")) -> (w313:T3)
              }
              frame Error {
                # "Resets the device with default values whenever there is an error"
                n104 = Unbundle By Name(w328) -> ("Source out"=w319:refnum<k15>, "Source channel name"=w317:string, "Load out"=w316:refnum<k15>, "Load channel name"=w315:string)
                n105 = call <instrlib>:"niDCPower Abort With Channels.vi"("error in (no error)"=w330, "channel name"=w315, "instrument handle"=w316) -> ("error out"=w323:errorcluster, "instrument handle out"=w320:refnum<k15>)  [unwired: 7 in]
                n106 = call <instrlib>:"niDCPower Reset With Channels.vi"("error in (no error)"=w323, "channel name"=w315, "instrument handle"=w320) -> ("error out"=w324:errorcluster, "instrument handle out"=w325:refnum<k15>)  [unwired: 7 in]
                n107 = call <instrlib>:"niDCPower Close.vi"("error in (no error)"=w324, "instrument handle"=w325) -> ("error out"=w318:errorcluster)  [unwired: 9 out]
                n108 = call <instrlib>:"niDCPower Abort With Channels.vi"("error in (no error)"=w318, "channel name"=w317, "instrument handle"=w319) -> ("error out"=w321:errorcluster, "instrument handle out"=w322:refnum<k15>)  [unwired: 7 in]
                n109 = call <instrlib>:"niDCPower Reset With Channels.vi"("error in (no error)"=w321, "channel name"=w317, "instrument handle"=w322) -> ("error out"=w327:errorcluster, "instrument handle out"=w326:refnum<k15>)  [unwired: 7 in]
                n110 = call <instrlib>:"niDCPower Close.vi"("error in (no error)"=w327, "instrument handle"=w326) -> ("error out"=w329:errorcluster)  [unwired: 9 out]
              }
            }
          }
        }
      }
    }
    frame "Power off the DUT" {
      # "Stops generation on the output channel and resets the channels to default values"
      n111 = Unbundle By Name(w350) -> ("Source resource name"=w352:string, "Load resource name"=w355:string)
      n112 = call <instrlib>:"niDCPower Initialize With Independent Channels.vi"("error in (no error)"=w362, "resource name"=w355) -> ("error out"=w356:errorcluster, "instrument handle out"=w354:refnum<k15>)  [unwired: 8 in]
      n113 = call-poly <instrlib>:"niDCPower Get Channel Name (Poly).vi"("error in (no error)"=w356, "index"="0", "instrument handle"=w354) -> ("error out"=w366:errorcluster, "name"=w363:string, "instrument handle out"=w364:refnum<k15>)  [unwired: 6 in]
      n114 = call <instrlib>:"niDCPower Configure Output Enabled.vi"("error in (no error)"=w366, "output enabled"=FALSE, "channel name"=w363, "instrument handle"=w364) -> ("error out"=w373:errorcluster, "instrument handle out"=w372:refnum<k15>)  [unwired: 6 in]
      n115 = call <instrlib>:"niDCPower Reset With Channels.vi"("error in (no error)"=w373, "channel name"=w363, "instrument handle"=w372) -> ("error out"=w367:errorcluster, "instrument handle out"=w368:refnum<k15>)  [unwired: 7 in]
      n116 = call <instrlib>:"niDCPower Close.vi"("error in (no error)"=w367, "instrument handle"=w368) -> ("error out"=w359:errorcluster)  [unwired: 9 out]
      n117 = call <instrlib>:"niDCPower Initialize With Independent Channels.vi"("error in (no error)"=w359, "resource name"=w352) -> ("error out"=w353:errorcluster, "instrument handle out"=w351:refnum<k15>)  [unwired: 8 in]
      n118 = call-poly <instrlib>:"niDCPower Get Channel Name (Poly).vi"("error in (no error)"=w353, "index"="0", "instrument handle"=w351) -> ("error out"=w358:errorcluster, "name"=w357:string, "instrument handle out"=w360:refnum<k15>)  [unwired: 6 in]
      n119 = call <instrlib>:"niDCPower Reset With Channels.vi"("error in (no error)"=w358, "channel name"=w357, "instrument handle"=w360) -> ("error out"=w370:errorcluster, "instrument handle out"=w369:refnum<k15>)  [unwired: 7 in]
      n120 = call <instrlib>:"niDCPower Close.vi"("error in (no error)"=w370, "instrument handle"=w369) -> ("error out"=w349:errorcluster)  [unwired: 9 out]
      n121 = Bundle By Name(cluster=w347, "Measurement Results.Status"="The DUT is powered OFF") -> (w345:T3)
    }
  }
  "error out" <- w2
  "measure call context out" <- w3
  n122 = Unbundle By Name(w1) -> ("Measurement Results"=→"measurement results":T1)
